vi "getProcessCommandEvent.vi"(11 "UserEvents in":refnum<class "UserEvents.lvclass">) -> (2 "ProcessCommandEvent":refnum<user-event>, 3 "UserEvents out":refnum<class "UserEvents.lvclass">)   [LabVIEW 2016, in "UserEvents.lvclass"]
uses:
  UserEvents.lvclass
  Types/ProcessCommandEvent.ctl
  Commands/Command/Command.lvclass
  UserEvents.lvclass/UserEvents.ctl
  Types/M1M3SupportTypes.lvlib
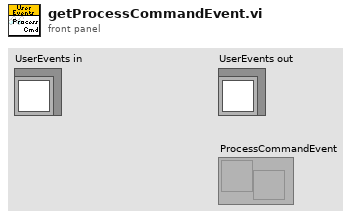
[diagram p1: front panel]
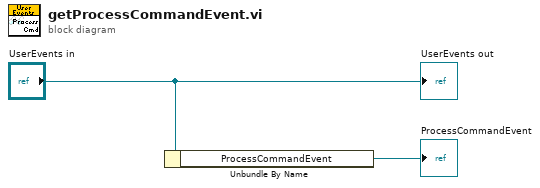
[diagram p0: block diagram]
diagram:
  n1 = Unbundle By Name("UserEvents in") -> ("ProcessCommandEvent"=→"ProcessCommandEvent":refnum<user-event>)
  "UserEvents out" <- "UserEvents in"
